vi "post_dust_event.vi"(7 "Small Accelerator?":bool, 8 "error in (no error)":errorcluster, 11 "Cluster":T1 {"File Location" items=["Currently Writing"=-3, "Labview Files"=-2, "Mars Data Processing Factility"=-1, "Local Cache "=0, "Old Storage"=1, "Storage"=2]; "Estimate Source" items=["Any Source."=-2, "No Shot"=-1, "Basic Labview Estimate"=0, "IDL Estimate From Andrew"=1, "IDL Estimate From Keith"=2, "Old Metadata"=3]}) -> (0 "error out":errorcluster, 1 "Experiment Settings":i32, 2 "Dust Event ID":i32, 3 "Test Server":bool)   [LabVIEW 2012]
uses:
  Public API/Post_Dust_Event.ctl
  Estimate_source.ctl
  File_location.ctl
  <vilib>/addons/database/Auxilliary.llb/DB Tools Cursor Type.ctl
  <vilib>/addons/database/Connection.llb/Conn Execute.vi
  <vilib>/addons/database/Recordset.llb/Rec Fetch Recordset Data (R).vi
  <vilib>/addons/database/Recordset.llb/Rec Destroy - Connection.vi
  <vilib>/addons/database/_DB Variant To Data/Database Variant To Data.xnode
  <vilib>/addons/database/NI_Database_API.lvlib
panel:
  # "Dust Event"
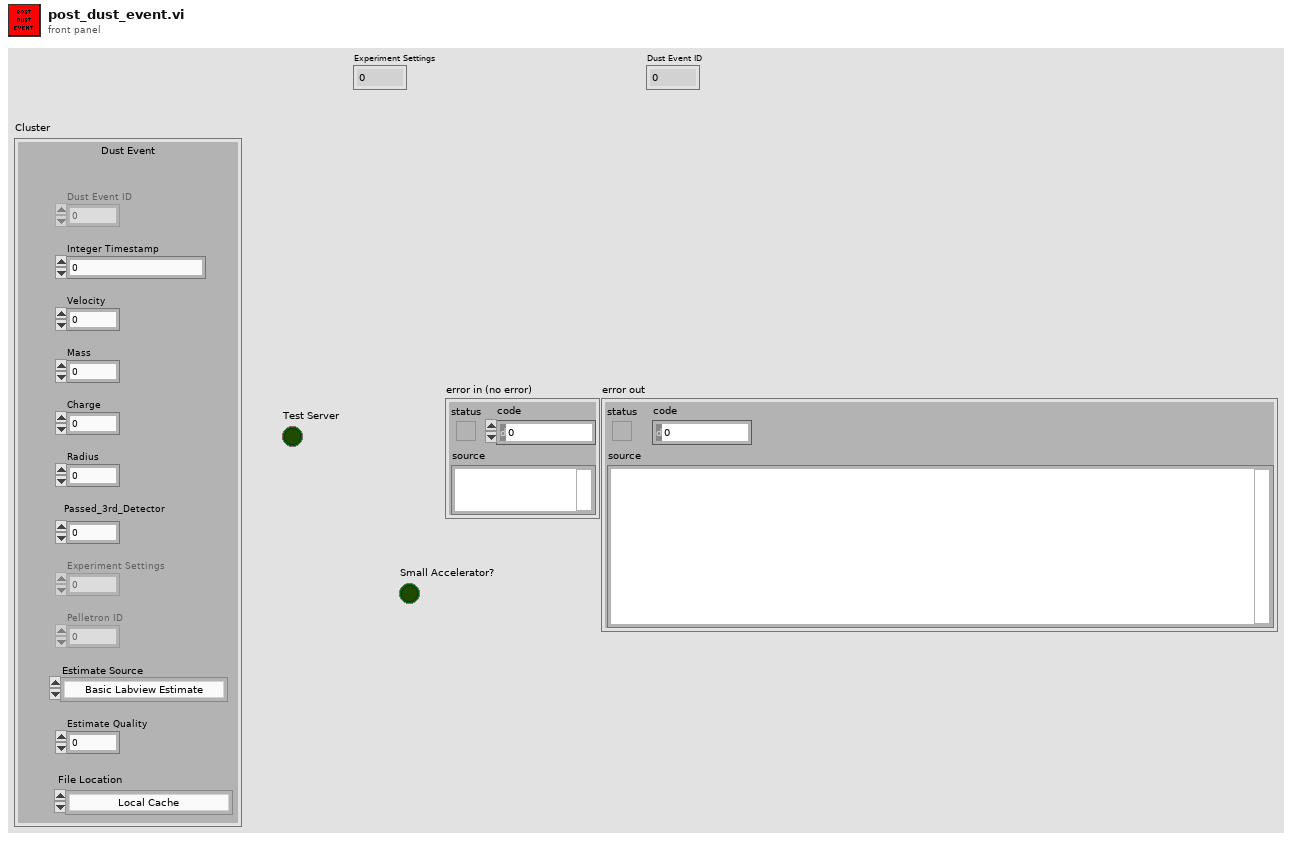
[diagram p1: front panel]
types:
  T1 = typedef "Post_Dust_Event.ctl" = cluster{"Dust Event ID":i64, "Integer Timestamp":i64, "Velocity":sgl, "Mass":sgl, "Charge":sgl, "Radius":sgl, "Passed_3rd_Detector":i8, "Experiment Settings":dbl, "Pelletron ID":i32, "Estimate Source":T2, "Estimate Quality":sgl, "File Location":T3, "id_dust_info":dbl}
  T2 = typedef "Estimate_source.ctl" = i8
  T3 = typedef "File_location.ctl" = i8
  T4 = typedef "NI_Database_API.lvlib/DB Tools Cursor Type.ctl" = enum16{"forward-only", "keyset", "dynamic", "static"}
  T5 = typedef "NI_Database_API.lvlib/Conn ObjectReference.ctl" = refnum<k1>
  T6 = typedef "NI_Database_API.lvlib/Rec ObjectReference.ctl" = refnum<k1>
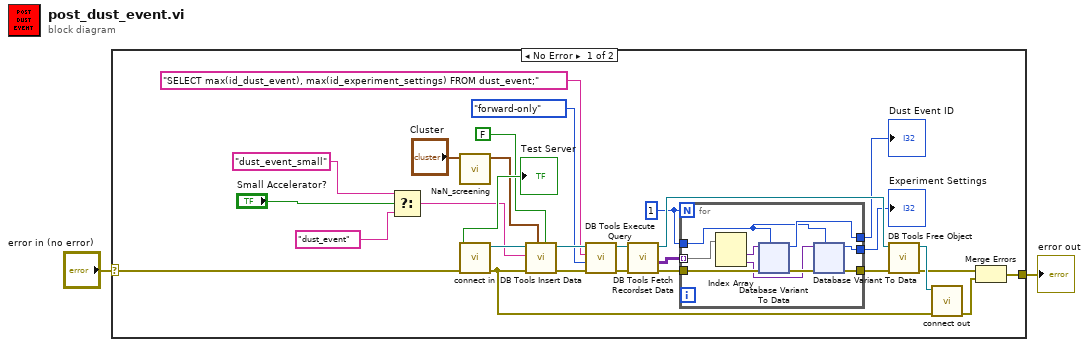
[diagram p0: block diagram]
diagram:
  n1 = case shown="No Error" "error in (no error)" {
    selector: "error in (no error)" -> [w27 w104]
    tunnel: [w24 w104] -> w1
    frame No Error {
      w14 = 1
      n2 = Select(t="dust_event_small" ("table"), s="Small Accelerator?", f="dust_event" ("table")) -> (s? t:f=w4:string)
      n3 = call "NaN_screening.vi"("Input"="Cluster") -> ("Output"=w9:T1)  [unwired: 10 in]
      n4 = call "connect in.vi"("error in (no error)"=w27) -> ("error out"=w26:errorcluster, "Database Connection"=w30:T5, "Test Server"=→"Test Server":bool)  [unwired: 6 in]
      n5 = call <vilib>:"DB Tools Insert Data.vi"("create table? (F)"=FALSE, "data"=w9, "error in (no error)"=w26, "table"=w4, "connection reference"=w30) -> ("error out"=w8:errorcluster, "connection reference out"=w21:T5)  [unwired: 5 in]
      n6 = call-poly <vilib>:"DB Tools Execute Query.vi"("error in (no error)"=w8, "cursor type"=DB_Tools_Cursor_Type."forward-only", "SQL query"="SELECT max(id_dust_event), max(id_experiment_settings) FROM dust_event;", "connection reference"=w21) -> ("error out"=w22:errorcluster, "recordset reference"=w23:T6)  [unwired: 4 in]
      n7 = call-poly <vilib>:"DB Tools Fetch Recordset Data.vi"("error in (no error)"=w22, "recordset reference"=w23) -> ("error out"=w12:errorcluster, "recordset data"=w15:variant[][], "recordset reference out"=w20:T6)  [unwired: 3 in]
      n8 = for {
        N: w14 -> [_]
        tunnel: w15 -> [w39] mode=indexing
        tunnel: w14 -> [w33]
        tunnel: [w37] -> w13
        tunnel: [w31] -> w11
        tunnel: w12 -> [w36]
        tunnel: [w32] -> w7
        n9 = Index Array(array=w39) -> (element #1=w38:variant, element #2=w34:variant)  [unwired: 2 in]
        n10 = xnode "Database Variant To Data"("database variant"=w38, "error in"=w36, "type"=w33) -> ("data"=w37:i32, "error out"=w35:errorcluster)
        n11 = xnode "Database Variant To Data"("database variant"=w34, "error in"=w35, "type"=w33) -> ("data"=w32:i32, "error out"=w31:errorcluster)
      }
      "Dust Event ID" <- w13
      "Experiment Settings" <- w7
      n12 = call-poly <vilib>:"DB Tools Free Object.vi"("error in (no error)"=w11, "recordset reference"=w20) -> ("error out"=w18:errorcluster, "connection reference"=w19:T5)  [unwired: 8 in]
      n13 = call "connect out.vi"("error in (no error)"=w26, "connection reference"=w19) -> ("error out"=w25:errorcluster)  [unwired: 9 in]
      n14 = Merge Errors(w18, w25) -> (w24:errorcluster)
    }
    frame Error {
    }
  }
  "error out" <- w1
